vi "Find Linespaces.vi"(8 "error in (no error)":errorcluster) -> (0 "error out":errorcluster, 3 "Rows where whitespace starts":i32[](array[numeric]))   [LabVIEW 2018, in "Image Management.lvlib"]
uses:
  Image Management.lvlib
  Action.ctl
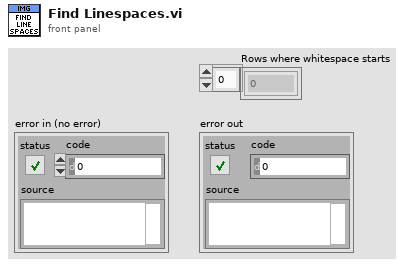
[diagram p1: front panel]
types:
  T1 = typedef "Image Management.lvlib/Action.ctl" = enum16{"Init", "Output Image Path", "Open Image in Default Program", "Find Linespaces", "Get Image Size (pixels)", "Close"}
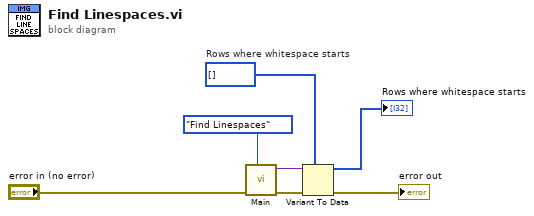
[diagram p0: block diagram]
diagram:
  w3 = i32[] []  # Rows where whitespace starts
  n1 = call "Main.vi"("Action"=Action."Find Linespaces", "Error In"="error in (no error)") -> ("Error Out"=w6:errorcluster, "Output"=w2:variant)  [unwired: 8 in]
  n2 = Variant To Data(error in=w6, type=w3, Variant=w2) -> (data=→"Rows where whitespace starts":i32[], error out=→"error out":errorcluster)
